vi "v1.8 2d array with time taking averages.vi"() -> ()   [LabVIEW 2018]
uses:
  <vilib>/DAQmx/read.llb/DAQmx Read (Analog 1D DBL NChan 1Samp).vi
  <vilib>/DAQmx/create/channels.llb/DAQmx Create Channel (AI-Voltage-Basic).vi
  <vilib>/DAQmx/configure/timing.llb/DAQmx Timing (Sample Clock).vi
  <vilib>/DAQmx/miscellaneous.llb/DAQmx Fill In Error Info.vi
  <vilib>/Analysis/baseanly.llb/Mean (DBL).vi
  <vilib>/Analysis/NI_AALBase.lvlib
panel:
  in  "stop 2":bool
  in  "stop":bool
  in  "Avg Of?":dbl
  in  "Record?":bool
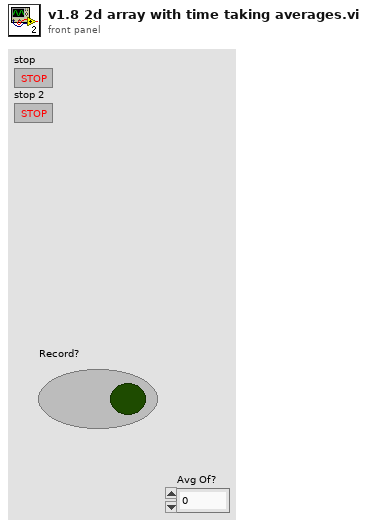
[diagram p1: front panel]
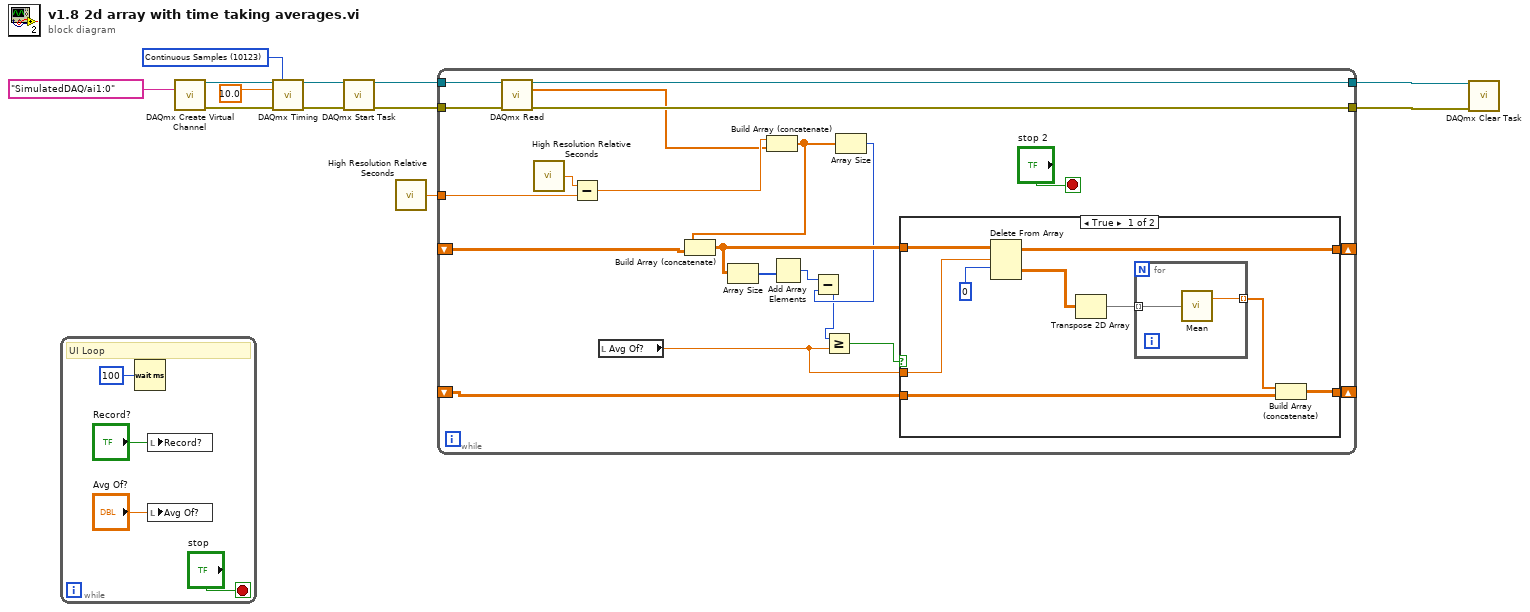
[diagram p0: block diagram]
diagram:
  w8 = 10123 items=["Finite Samples"=10178, "Continuous Samples"=10123, "Hardware Timed Single Point"=12522] ("sample mode")
  n1 = while {
    stop <- "stop" stop-if-true
    # "UI Loop"
    n2 = Wait (ms)(milliseconds to wait=u32 100) -> ()  [unwired: 1 out]
    n3 = local write "Record?"("Record?") -> ()
    n4 = local write "Avg Of?"("Avg Of?") -> ()
  }
  n5 = call-poly <vilib>:"DAQmx Create Virtual Channel.vi"("physical channels"=tag "SimulatedDAQ/ai1:0") -> ("task out"=w9:refnum<k21>, "error out"=w10:errorcluster)  [unwired: 13 in]
  n6 = call-poly <vilib>:"DAQmx Timing.vi"("task/channels in"=w9, "sample mode"=w8, "rate"=10.0, "error in"=w10) -> ("task out"=w11:refnum<k21>, "error out"=w12:errorcluster)  [unwired: 10 in]
  n7 = call <vilib>:"DAQmx Start Task.vi"("task/channels in"=w11, "error in"=w12) -> ("task out"=w2:refnum<k21>, "error out"=w3:errorcluster)  [unwired: 12 in]
  n8 = call <vilib>:"High Resolution Relative Seconds.vi"() -> ("relative seconds"=w1:dbl)
  n9 = while {
    tunnel: w2 -> [w34]
    tunnel: w3 -> [w37]
    tunnel: [w36] -> w6
    tunnel: [w35] -> w5
    tunnel: w1 -> [w31]
    shift-right: [w28] -> _
    shift-left: _ -> [w27]
    shift-right: [w18] -> _
    shift-left: _ -> [w17]
    stop <- "stop 2" stop-if-true
    # "Aquisition Loop"
    n10 = call-poly <vilib>:"DAQmx Read.vi"("task/channels in"=w34, "error in"=w37) -> ("task out"=w36:refnum<k21>, "data"=w29:dbl[], "error out"=w35:errorcluster)  [unwired: 11 in]
    n11 = call <vilib>:"High Resolution Relative Seconds.vi"() -> ("relative seconds"=w32:dbl)
    n12 = Subtract(x=w32, y=w31) -> (x-y=w30:dbl)
    n13 = local read "Avg Of?"() -> (w19:dbl)
    n14 = Build Array (concatenate)(w30, w29) -> (w26:dbl[])
    n15 = Build Array (concatenate)(w26, w27) -> (w25:dbl[][])
    n16 = Array Size(array=w25) -> (size(s)=w24:i32[])
    n17 = Add Array Elements(numeric array=w24) -> (sum=w23:i32)
    n18 = Array Size(array=w26) -> (size(s)=w22:i32)
    n19 = Subtract(x=w23, y=w22) -> (x-y=w20:i32)
    n20 = Greater Or Equal?(x=w20, y=w19) -> (x >= y?=w21:bool)
    n21 = case shown="True" w21 {
      tunnel: [w43 w50] -> w28
      tunnel: w25 -> [w46 w50]
      tunnel: w19 -> [w45 _]
      tunnel: [w39 w49] -> w18
      tunnel: w17 -> [w38 w49]
      frame True {
        n22 = Delete From Array(array=w46, length=w45, index (row)=0) -> (deleted portion=w42:dbl[][], array with subset deleted=w43:dbl[][])  [unwired: 1 in]
        n23 = Transpose 2D Array(2D array=w42) -> (transposed array=w41:dbl[][])
        n24 = for {
          tunnel: w41 -> [w48] mode=indexing
          tunnel: [w47] -> w40 mode=indexing
          n25 = call-poly <vilib>:"Mean.vi"("X"=w48) -> ("mean"=w47:dbl)  [unwired: 1 out]
        }
        n26 = Build Array (concatenate)(w40, w38) -> (w39:dbl[][])
      }
      frame False {
      }
    }
  }
  n27 = call <vilib>:"DAQmx Clear Task.vi"("task in"=w6, "error in"=w5) -> ()  [unwired: 13 in, 1 out]
